vi "Service Stop Handler.vi"(8 "error in":errorcluster, 9 "stop server user event":T1, 10 "stop button ref":refnum<vi>, 11 "measurement service v1 in":refnum<class "Measurement Service V1.lvclass">) -> (0 "error out":errorcluster, 3 "measurement service v1 out":refnum<class "Measurement Service V1.lvclass">)   [LabVIEW 2020, in "Measurement Plugin Measurement Server.lvlib" / "Measurement Service V1.lvclass"]
uses:
  Measurement Service V1.lvclass
  Helpers/TypeDefs/Stop Server User Event.ctl
  Measurement Service V1.lvclass/Measurement Service V1.ctl
  gRPC/Generated APIs/ni/measurementlink/measurement/v1/RPC Service/MeasurementService/MeasurementServiceBaseV1.lvclass
  C:/Program Files/National Instruments/LabVIEW 2020/vi.lib/gRPC/LabVIEW gRPC Servicer/ServiceBase/ServiceBase.lvclass
  IMeasurement Service/IMeasurement Service.lvclass
  Measurement Plugin Measurement Server.lvlib
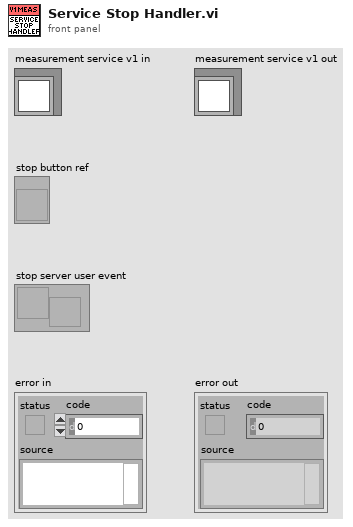
[diagram p1: front panel]
types:
  T1 = typedef "Measurement Plugin Measurement Server.lvlib/Stop Server User Event.ctl" = refnum<user-event>
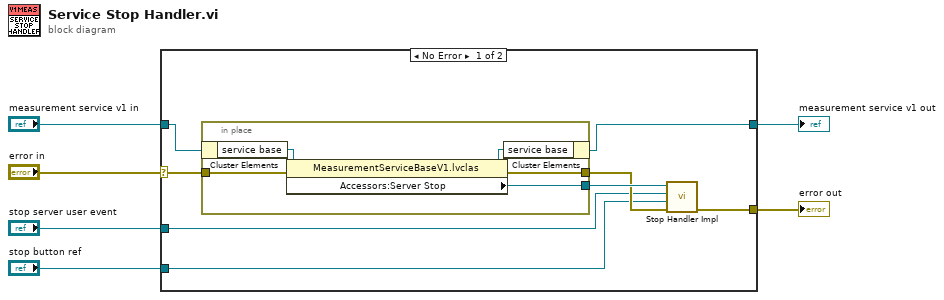
[diagram p0: block diagram]
diagram:
  n1 = case shown="No Error" "error in" {
    selector: "error in" -> [w13 w21]
    tunnel: [w12 w21] -> w5
    tunnel: [w11 w20] -> w3
    tunnel: "measurement service v1 in" -> [w14 w20]
    tunnel: "stop button ref" -> [w8 _]
    tunnel: "stop server user event" -> [w7 _]
    frame No Error {
      n2 = in-place {
        in-place-border: [w17] -> w10
        in-place-border: w13 -> [w16]
        in-place-border: [w15] -> w9
        n3 = in-place-cluster #1(w14) -> ("service base"=w19:refnum<class "MeasurementServiceBaseV1.lvclass">)
        n4 = property class="MeasurementServiceBaseV1.lvclas"(reference=w19, error in=w16) -> (reference out=w18:refnum<class "MeasurementServiceBaseV1.lvclass">, error out=w15:errorcluster, "Accessors:Server Stop"=w17:refnum<user-event>)
        n5 = in-place-cluster #1("service base"=w18) -> (w11:refnum<class "Measurement Service V1.lvclass">)
      }
      n6 = call "Stop Handler Impl.vi"("error in"=w9, "stop button ref"=w8, "stop server user event"=w7, "stop server broadcast event"=w10) -> ("error out"=w12:errorcluster)  [unwired: 7 in]
    }
    frame Error {
    }
  }
  "error out" <- w5
  "measurement service v1 out" <- w3
